vi "C2F.vi"() -> ()   [LabVIEW 2021]
panel:
  out "Fahrenheit":dbl
  in  "Celsius":dbl
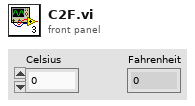
[diagram p1: front panel]
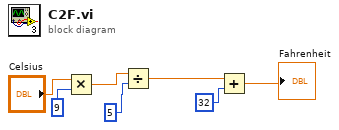
[diagram p0: block diagram]
diagram:
  n1 = Multiply(x="Celsius", y=9) -> (x*y=w2:dbl)
  n2 = Divide(x=w2, y=5) -> (x/y=w1:dbl)
  n3 = Add(x=w1, y=32) -> (x+y=→"Fahrenheit":dbl)
